vi "createRuntimeMenu.vi"(8 "error in (no error)":errorcluster, 10 "menu reference":refnum<k9>, 11 "QControl_Graph in":refnum<class "QControl_Graph.lvclass">) -> (0 "error out":errorcluster, 3 "QControl_Graph out":refnum<class "QControl_Graph.lvclass">)   [LabVIEW 2017, in "QControl_Graph.lvclass"]
uses:
  QControl_Graph.lvclass
  C:/Program Files (x86)/National Instruments/LabVIEW 2017/vi.lib/QSI/QControls/QControl Classes/Control/Control.lvclass
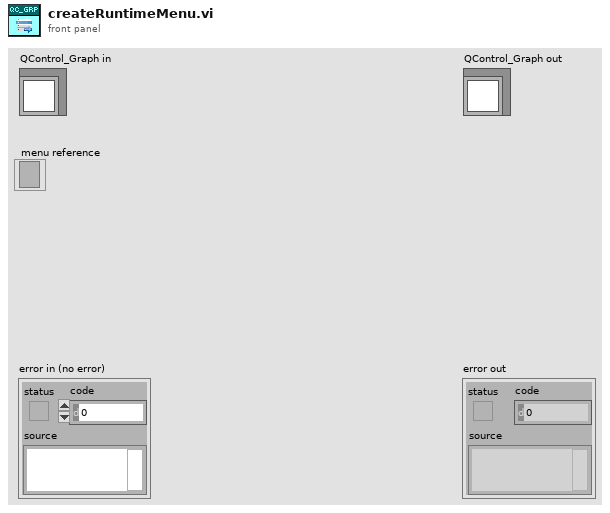
[diagram p1: front panel]
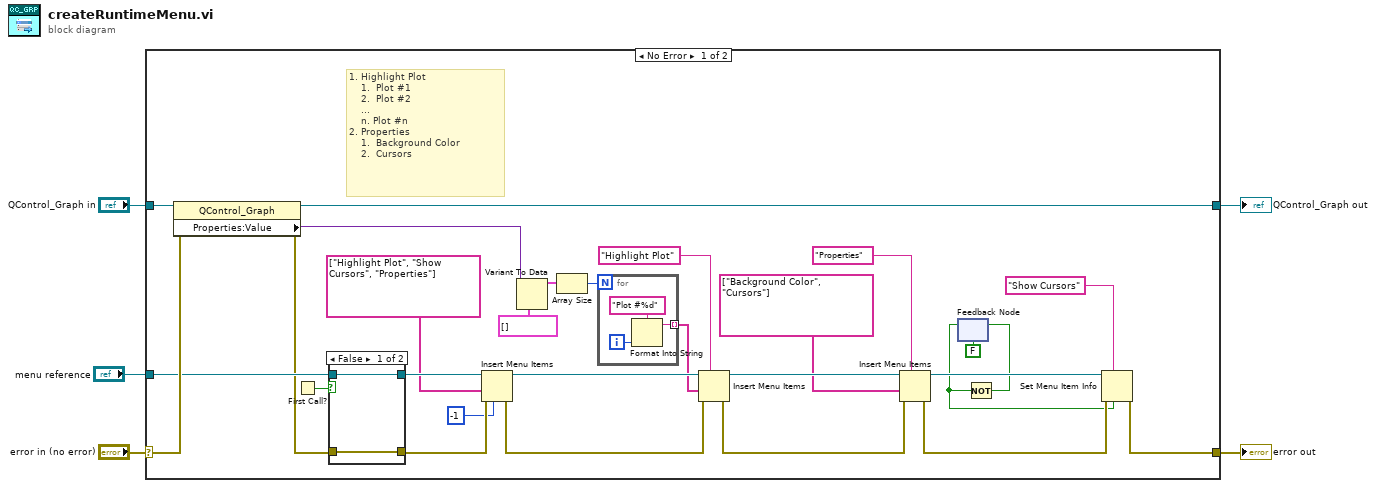
[diagram p0: block diagram]
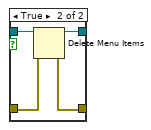
[diagram p2: hidden frame]
diagram:
  n1 = case shown="No Error" "error in (no error)" {
    selector: "error in (no error)" -> [w33 w45]
    tunnel: [w12 w45] -> w4
    tunnel: [w32 w44] -> w2
    tunnel: "QControl_Graph in" -> [w34 w44]
    tunnel: "menu reference" -> [w31 _]
    frame No Error {
      # "1. Highlight Plot\n    1.  Plot #1\n    2.  Plot #2\n    ...\n    n. Plot #n\n2. Properties\n    1.  Background Color\n    2.  Cursors"
      n2 = property class="QControl_Graph"(reference=w34, error in=w33) -> (reference out=w32:refnum<class "QControl_Graph.lvclass">, error out=w25:errorcluster, "Properties:Value"=w22:variant)
      n3 = First Call?() -> (First Call?: T/F=w11:bool)
      n4 = case shown="False" w11 {
        tunnel: w31 -> [w36 w40]
        tunnel: [w36 w39] -> w30
        tunnel: [w35 w38] -> w28
        tunnel: w25 -> [w35 w37]
        frame False {
        }
        frame True {
          n5 = Delete Menu Items(6:w37, 9:w40) -> (0:w38:errorcluster, 3:w39:refnum<k9>)  [unwired: 2 in]
        }
      }
      n6 = Insert Menu Items(4:-1, 6:w28, 7:string[] ["Highlight Plot", "Show Cursors", "Properties"] ("item tags"), 9:w30) -> (0:w27:errorcluster, 3:w29:refnum<k9>)  [unwired: 2 in, 1 out]
      n7 = Variant To Data(type=cluster{dbl[], dbl[]}[] [], Variant=w22) -> (data=w21:cluster{dbl[], dbl[]}[])  [unwired: 1 in, 1 out]
      n8 = Array Size(array=w21) -> (size(s)=w20:i32)
      n9 = for {
        N: w20 -> [_]
        tunnel: [w41] -> w18 mode=indexing
        i -> [w43]
        n10 = Format Into String(format string="Plot #%d", w43) -> (resulting string=w41:string)  [unwired: 2 in, 1 out]
      }
      n11 = Insert Menu Items(5:"Highlight Plot", 6:w27, 7:w18, 9:w29) -> (0:w14:errorcluster, 3:w17:refnum<k9>)  [unwired: 2 in, 1 out]
      n12 = Insert Menu Items(5:"Properties", 6:w14, 7:string[] ["Background Color", "Cursors"] ("item tags"), 9:w17) -> (0:w9:errorcluster, 3:w10:refnum<k9>)  [unwired: 2 in, 1 out]
      n13 = feedback #1(FALSE) -> (w7:bool)
      n14 = Not(x=w7) -> (.not. x?=w6:bool)
      n15 = feedback-in #1(w6) -> ()
      n16 = Set Menu Item Info(6:w7, 7:"Show Cursors", 8:w9, 11:w10) -> (0:w12:errorcluster)  [unwired: 3 in, 1 out]
    }
    frame Error {
    }
  }
  "error out" <- w4
  "QControl_Graph out" <- w2
